vi "Set_EU.vi"(0 "reference in":refnum<class "Sig_Digital.lvclass">, 5 "EU":bool, 11 "error in (no error)":errorcluster) -> (4 "reference out":refnum<class "Sig_Digital.lvclass">, 15 "error out":errorcluster)   [LabVIEW 2019, in "Sig_Digital.lvclass"]
uses:
  Sig_Digital.lvclass
  D:/GIT H4000/H4000/src/Proccess_class/Proccess.lvclass
  Sig_Digital.lvclass/Sig_Digital.ctl
  Proccess_class/Proccess.lvclass/Proccess.ctl
  Proccess_class/Read TagName.vi
  Proccess_class/Read Logger.vi
  Logger_class/WriteEvent.vi
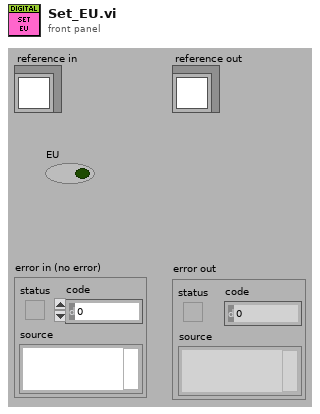
[diagram p1: front panel]
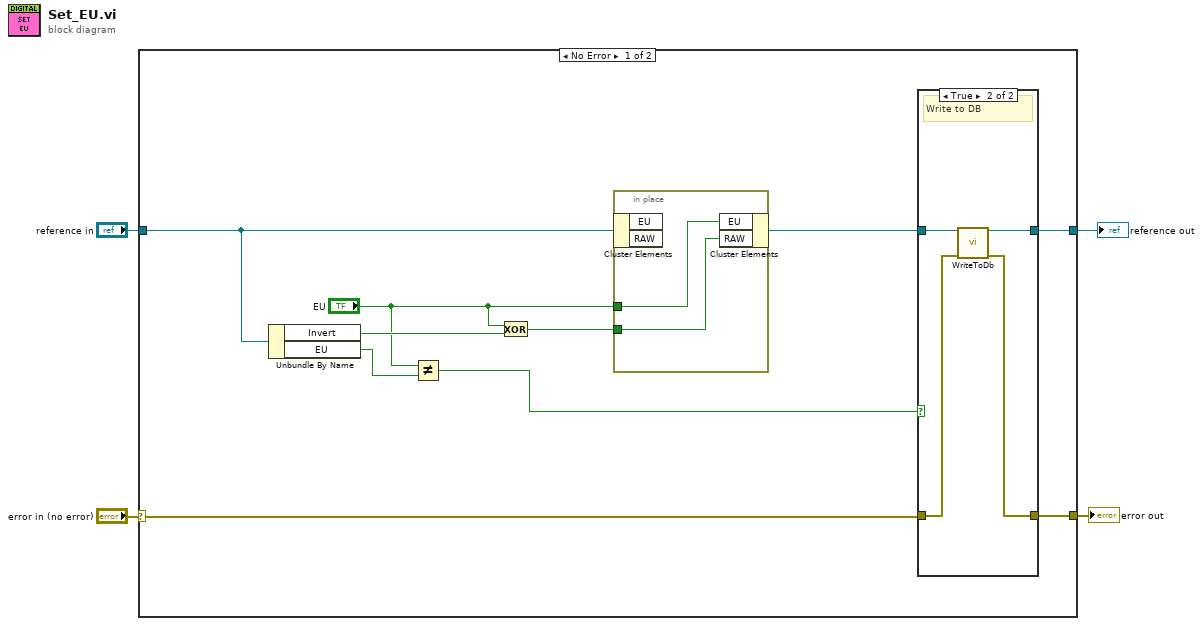
[diagram p0: block diagram]
diagram:
  n1 = case shown="No Error" "error in (no error)" {
    selector: "error in (no error)" -> [w14 w24]
    tunnel: [w9 w24] -> w3
    tunnel: [w8 w23] -> w1
    tunnel: "reference in" -> [w7 w23]
    frame No Error {
      n2 = Unbundle By Name(w7) -> ("Invert"=w13:bool, "EU"=w11:bool)
      n3 = Not Equal?(x="EU", y=w11) -> (x != y?=w10:bool)
      n4 = Exclusive Or(1:w13, 2:"EU") -> (0:w6:bool)
      n5 = in-place {
        in-place-border: "EU" -> [w16]
        in-place-border: w6 -> [w15]
        n6 = in-place-cluster #1(w7) -> ()  [unwired: 2 out]
        n7 = in-place-cluster #1("EU"=w16, "RAW"=w15) -> (w5:refnum<class "Sig_Digital.lvclass">)
      }
      n8 = case shown="True" w10 {
        tunnel: w5 -> [w18 w21]
        tunnel: [w18 w20] -> w8
        tunnel: w14 -> [w17 w22]
        tunnel: [w17 w19] -> w9
        frame False {
        }
        frame True {
          # "Write to DB"
          n9 = call "WriteToDb.vi"("reference in"=w21, "error in (no error)"=w22) -> ("reference out"=w20:refnum<class "Sig_Digital.lvclass">, "error out"=w19:errorcluster)  [unwired: 12 in]
        }
      }
    }
    frame Error {
    }
  }
  "error out" <- w3
  "reference out" <- w1
